vi "Config Brightness.vi"(8 "error in":errorcluster, 10 "Brightness (5)":i32=5 max=9, 11 "VISA resource name":refnum<visa-resource-name>) -> (0 "error out":errorcluster, 3 "VISA resource name out":refnum<visa-resource-name>)   [LabVIEW 2016, in "Andeen-Hagerling 2550.lvlib"]
doc: "This VI sets the overall brightness of all of the front panel displays."
uses:
  Andeen-Hagerling 2550.lvlib
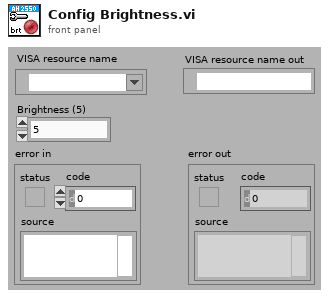
[diagram p1: front panel]
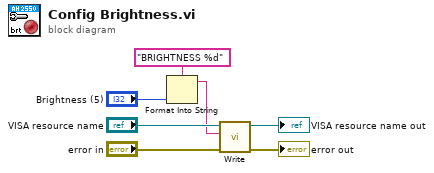
[diagram p0: block diagram]
diagram:
  n1 = Format Into String(format string="BRIGHTNESS %d", "Brightness (5)") -> (resulting string=w1:string)  [unwired: 2 in, 1 out]
  n2 = call "Write.vi"("error in"="error in", "command"=w1, "VISA resource name"="VISA resource name") -> ("error out"=→"error out":errorcluster, "VISA resource name out"=→"VISA resource name out":refnum<visa-resource-name>)  [unwired: 7 in]
